vi "Decode Points Referee.vi"(7 "Boolean":bool=TRUE, 8 "error in":errorcluster, 9 "array":u8[](array[numeric]), 10 "Key":i32=5) -> (0 "error out":errorcluster, 1 "array w/ subset deleted out":u8[](array[numeric]), 3 "Point":cluster{"x":sgl, "y":sgl})   [LabVIEW 2020]
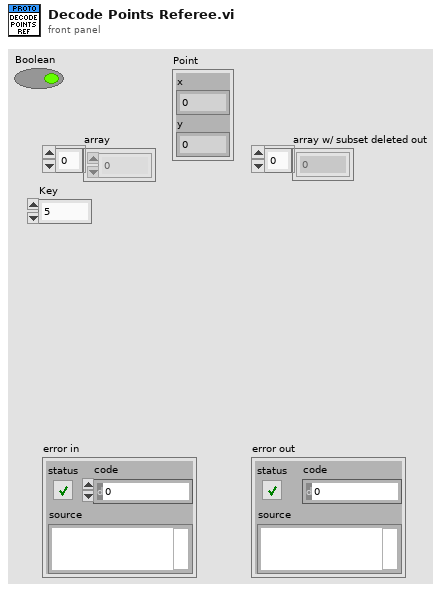
[diagram p1: front panel]
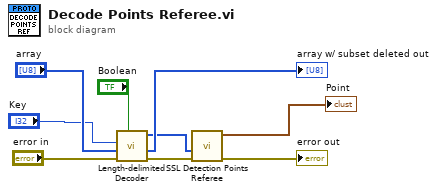
[diagram p0: block diagram]
diagram:
  n1 = call "Length-delimited Decoder.vi"("Optional"="Boolean", "error in (no error)"="error in", "Array"="array", "Key"="Key") -> ("error out"=w2:errorcluster, "array w/ subset deleted"=→"array w/ subset deleted out":u8[], "Length-delimited"=w3:u8[])  [unwired: 4 in, 1 out]
  n2 = call "SSL Detection Points Referee.vi"("error in"=w2, "Array"=w3) -> ("error out"=→"error out":errorcluster, "Point"=→"Point":cluster{"x":sgl, "y":sgl})  [unwired: 7 in, 1 out]
